vi "SECoP_dataFindStructIndex.vi"(7 "Position":u32, 8 "error in (no error)":errorcluster, 9 "struct_name":string, 10 "SECoP_dataPtr":T1 {"ptr64" format="%.0x"; "ptr32" format="%.0x"}, 11 "DLL path (in)":T2) -> (0 "error out":errorcluster, 2 "index":u32, 3 "DLL path (out)":T2)   [LabVIEW 2015, in "SECoP.lvlib"]
doc: "Call <b>\"SECoP_dataFindStructIndex.vi\"</b> to find the index of named struct item of a complex data type.\n\n<b>DLL path</b> input and output of cluster from \"SECoP-Initialize.vi\"\n<b>SECoP_dataPtr</b> data to access\n<b>Position</b> points to a virtual flattened entry of the data type; for a top level struct use 0\n<b>struct_name</b> name of the requested struct item\n<b>index</b> found position of the requested struct item for direct access with <b>\"SECoP_data*.vi\"</b>"
uses:
  SECoP.lvlib
  SECoP-data.ctl
  SECoP-libraries.ctl
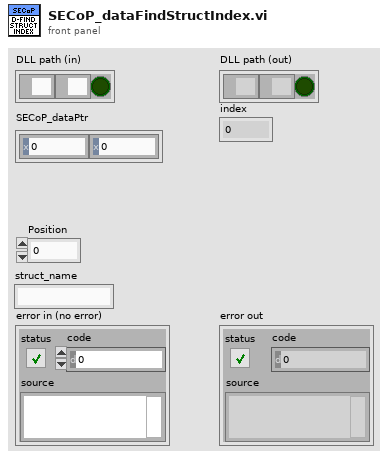
[diagram p1: front panel]
types:
  T1 = typedef "SECoP.lvlib/SECoP-data.ctl" = cluster{"ptr32":u32, "ptr64":u64}
  T2 = typedef "SECoP.lvlib/SECoP-libraries.ctl" = cluster{"serverDLL":path, "variantDLL":path, "cleanup_mode":bool}
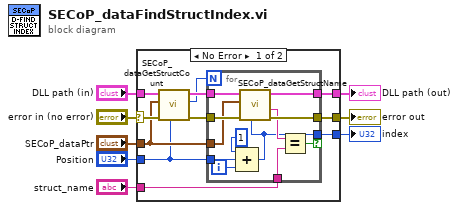
[diagram p0: block diagram]
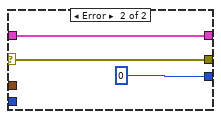
[diagram p2: hidden frame]
diagram:
  n1 = case shown="No Error" "error in (no error)" {
    selector: "error in (no error)" -> [w19 w33]
    tunnel: "DLL path (in)" -> [w18 w34]
    tunnel: [w12 w34] -> w2
    tunnel: [w11 w33] -> w3
    tunnel: "Position" -> [w9 _]
    tunnel: [w10 u32 0] -> w4
    tunnel: "SECoP_dataPtr" -> [w14 _]
    tunnel: "struct_name" -> [w13 _]
    frame No Error {
      n2 = call "SECoP_dataGetStructCount.vi"("Position"=w9, "error in (no error)"=w19, "SECoP_dataPtr"=w14, "DLL path (in)"=w18) -> ("error out"=w16:errorcluster, "no. of struct elements"=w15:u32, "DLL path (out)"=w17:T2)  [unwired: 5 in]
      n3 = for {
        N: w15 -> [_]
        tunnel: w17 -> [w31]
        tunnel: w16 -> [w30]
        tunnel: w14 -> [w29]
        tunnel: [w20] -> w10 if=w25
        tunnel: w13 -> [w26]
        tunnel: [w28] -> w12
        tunnel: [w27] -> w11
        tunnel: w9 -> [w22]
        i -> [w23]
        n4 = Compound Arithmetic op=ADD(u32 1, w22, w23) -> (w20:u32)
        n5 = call "SECoP_dataGetStructName.vi"("Position"=w20, "error in (no error)"=w30, "SECoP_dataPtr in"=w29, "DLL path (in)"=w31) -> ("error out"=w27:errorcluster, "struct_name"=w24:string, "DLL path (out)"=w28:T2)  [unwired: 5 in]
        n6 = Equal?(x=w24, y=w26) -> (x = y?=w25:bool)
      }
    }
    frame Error {
    }
  }
  "DLL path (out)" <- w2
  "error out" <- w3
  "index" <- w4
